vi "Insight_RW_Fixed_Wavelength_Delay.vi"(7 "Parameter Type":enum16{"Value", "MAXimum", "MINimum", "DEFault"}(ring), 8 "error in (no error)":errorcluster, 9 "Mode (Read / Write)":enum8{"Write", "Read"}(ring), 10 "Delay (usec)":dbl, 11 "telnet connection":T1) -> (0 "error out":errorcluster, 1 "response data":string, 2 "Delay (usec) ?":dbl, 3 "telnet  connection out":T1)   [LabVIEW 2011]
doc: "Insight Photonic Solutions\n\nThis reads or write the delay for the Wavelength Ready trigger that is generated each time a new fixed wavelength value is set. Wavelength Ready trigger is emitted from the Data Valid Trigger output. Use this trigger as a hardware signal that the laser has reached the desired wavelength\n\nInputs:\nRead/Write : command or query the delay of the Wavelength Ready Trigger.\nParameter Type - Tells the VI whether the command should use a Value or a keyword MAXimum, MINimum or DEFault to set the parameter value. (Default = Value).\nDelay (usec): specify to within 1 usec precision, up to 100,000 usec (100 msec).\n\nOutputs:\nResponse Data - Entire string response from the laser.\nDelay (usec)? -delay time, in usec, parsed from the total string response.\n\nver 1.0 - original release\nver 3.3 - changed parser to handle responses from pre and post version 3.3 of Atlas\nver 3.4 - accepts key word values Max, Min or Default in addition to numeric values of the parameter"
uses:
  Telnet Session.ctl
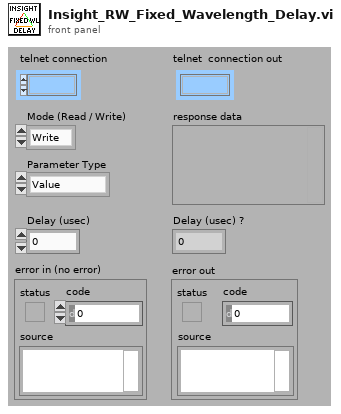
[diagram p1: front panel]
types:
  T1 = typedef "Telnet Session.ctl" = refnum<k1>
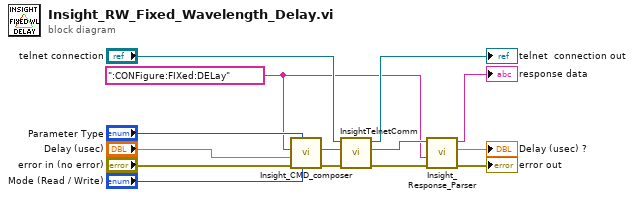
[diagram p0: block diagram]
diagram:
  w4 = ":CONFigure:FIXed:DELay" ("String")
  n1 = call "Insight_CMD_composer.vi"("Mode (Read / Write)"="Mode (Read / Write)", "Parameter Type"="Parameter Type", "error in (no error)"="error in (no error)", "Value"="Delay (usec)", "CMD"=w4) -> ("error out"=w7:errorcluster, "Command String"=w6:string)  [unwired: 5 in]
  n2 = call "InsightTelnetComm.vi"("error in"=w7, "write buffer (\"\")"=w6, "telnet connection"="telnet connection") -> ("error out"=w12:errorcluster, "response data"=w8:string, "telnet  connection out"=→"telnet  connection out":T1)  [unwired: 4 in]
  n3 = call "Insight_Response_Parser.vi"("error in (no error)"=w12, "Command String"=w4, "Laser Response In"=w8) -> ("error out"=→"error out":errorcluster, "Value"=→"Delay (usec) ?":dbl, "Laser Response Out"=→"response data":string)  [unwired: 6 in]
